vi "deregister.vi"(0 "HGF_SVMonitor":refnum<class "HGF_SVMonitor.lvclass">, 1 "SV":string, 2 "HGF_NetworkVisitor":refnum<class "HGF_NetworkVisitor.lvclass">, 3 "HGF_TriggeredEvent":refnum<class "HGF_TriggeredEvent.lvclass">, 4 "Rem SV/Visitor from List":bool, 5 "error in (no error)":errorcluster) -> (14 "HGF_SVMonitor":refnum<class "HGF_SVMonitor.lvclass">, 19 "error out":errorcluster)   [LabVIEW 2012, in "HGF_SV.lvlib" / "HGF_SVMonitor.lvclass"]
uses:
  HGF_SVMonitor.lvclass
  HGF_BaseClasses/HGF_TriggeredEvent/HGF_TriggeredEvent.lvclass
  HGF_BaseClasses/HGF_NetworkVisitor/HGF_NetworkVisitor.lvclass
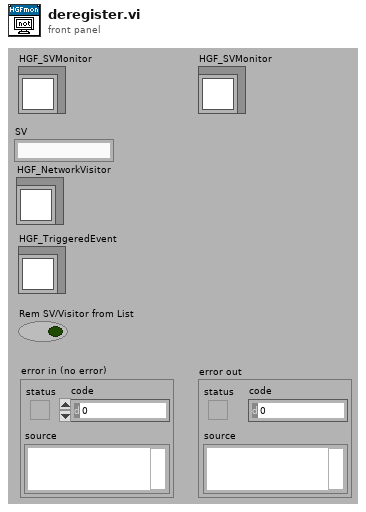
[diagram p1: front panel]
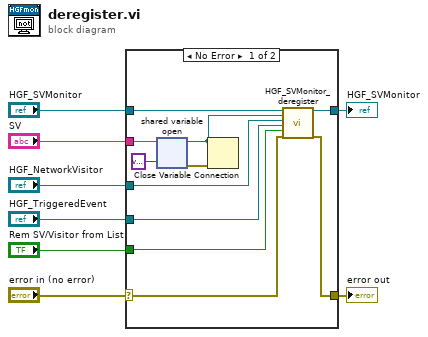
[diagram p0: block diagram]
diagram:
  n1 = case shown="No Error" "error in (no error)" {
    selector: "error in (no error)" -> [w16 w20]
    tunnel: [w15 w20] -> w7
    tunnel: "HGF_SVMonitor" -> [w19 w21]
    tunnel: [w18 w21] -> w5
    tunnel: "Rem SV/Visitor from List" -> [w17 _]
    tunnel: "HGF_TriggeredEvent" -> [w14 _]
    tunnel: "HGF_NetworkVisitor" -> [w13 _]
    tunnel: "SV" -> [w10 _]
    frame No Error {
      n2 = shared-variable-open(w10, variant ("variant")) -> (w11:refnum<k21>, w9:errorcluster)  [unwired: 2 in]
      n3 = Close Variable Connection(8:w9, 11:w11) -> ()  [unwired: 1 out]
      n4 = call "HGF_SVMonitor_deregister.vi"("HGF_SVMonitor in"=w19, "shared variable refnum"=w11, "HGF_NetworkVisitor"=w13, "HGF_TriggeredEvent"=w14, "Rem SV/Visitor from List"=w17, "error in (no error)"=w16) -> ("HGF_SVMonitor out"=w18:refnum<class "HGF_SVMonitor.lvclass">, "error out"=w15:errorcluster)  [unwired: 12 in]
    }
    frame Error {
    }
  }
  "error out" <- w7
  "HGF_SVMonitor" <- w5
